vi "Setup Motors.vi"   [LabVIEW 2014]
uses:
  <vilib>/Rock Robotics/SystemInterfaces/DIO/FPGA_DIOPWMChannel.ctl
  <vilib>/Rock Robotics/SystemInterfaces/Typedef/FPGA_TypedefDigitalModule.ctl
  <vilib>/Rock Robotics/WPI/Joystick/WPI_JoystickDeviceEnum.ctl
  <vilib>/Rock Robotics/SystemInterfaces/Typedef/FPGA_TypedefAnalogModule.ctl
  <vilib>/Rock Robotics/SystemInterfaces/AI/FPGA_AIChannel.ctl
  <vilib>/Rock Robotics/WPI/Solenoid/WPI_SolenoidChannel.ctl
  <vilib>/Rock Robotics/SystemInterfaces/AI/FPGA_AIGyroChannel.ctl
  <vilib>/Rock Robotics/SystemInterfaces/Typedef/FPGA_TypedefAnalogModuleForGyro.ctl
  <vilib>/Rock Robotics/SystemInterfaces/DIO/FPGA_DIOChannel.ctl
  <vilib>/Rock Robotics/WPI/SafetyOutput/WPI_SafetyOutputConfigMenu.ctl
  <vilib>/Rock Robotics/WPI/MotorControl/WPI_MotorControlOpen Talon.vi
  <vilib>/Rock Robotics/WPI/Solenoid/WPI_SolenoidOpenSingle.vi
  <vilib>/Rock Robotics/WPI/Switch/WPI_SwitchOpenLimit.vi
  Global Variables.vi
types:
  T1 = typedef "WPI_SafetyOutputConfigMenu.ctl" = enum16{"Enable", "Disable"}
  T2 = typedef "FPGA_DIOChannel.ctl" = enum8{"DIO 0", "DIO 1", "DIO 2", "DIO 3", "DIO 4", "DIO 5", "DIO 6", "DIO 7", "DIO 8", "DIO 9", "DIO MXP 0", "DIO MXP 1", "DIO MXP 2", "DIO MXP 3", "DIO MXP 4", "DIO MXP 5", "DIO MXP 6", "DIO MXP 7", "DIO MXP 8", "DIO MXP 9", "DIO MXP 10", "DIO MXP 11", "DIO MXP 12", "DIO MXP 13", "DIO MXP 14", "DIO MXP 15", "Invalid"}
  T3 = typedef "FPGA_TypedefDigitalModule.ctl" = enum16{"Controller 1"}
  T4 = typedef "FPGA_TypedefAnalogModuleForGyro.ctl" = enum16{"Controller 1"}
  T5 = typedef "FPGA_AIGyroChannel.ctl" = enum8{"AI 0", "AI 1", "Invalid"}
  T6 = typedef "WPI_SolenoidChannel.ctl" = enum8{"Solenoid 0", "Solenoid 1", "Solenoid 2", "Solenoid 3", "Solenoid 4", "Solenoid 5", "Solenoid 6", "Solenoid 7", "Invalid"}
  T7 = typedef "FPGA_DIOPWMChannel.ctl" = enum8{"PWM 0", "PWM 1", "PWM 2", "PWM 3", "PWM 4", "PWM 5", "PWM 6", "PWM 7", "PWM 8", "PWM 9", "PWM MXP 0", "PWM MXP 1", "PWM MXP 2", "PWM MXP 3", "PWM MXP 4", "PWM MXP 5", "PWM MXP 6", "PWM MXP 7", "PWM MXP 8", "PWM MXP 9", "Invalid"}
  T8 = typedef "FPGA_AIChannel.ctl" = enum8{"AI 0", "AI 1", "AI 2", "AI 3", "AI MXP 0", "AI MXP 1", "AI MXP 2", "AI MXP 3", "Invalid"}
  T9 = typedef "FPGA_TypedefAnalogModule.ctl" = enum16{"Controller 1"}
  T10 = typedef "WPI_JoystickDeviceEnum.ctl" = enum16{"USB 0", "USB 1", "USB 2", "USB 3", "USB 4", "USB 5"}
  T11 = typedef "WPI_MotorControlDeviceRef.ctl" = cluster{"DeviceStatus":errorcluster, "Type":T12, "PWM":cluster{"Controller":T3, "PWM Channel":T7, "DeadBand":T13}, "CAN":cluster{"Device Number":u8, "Control Mode":T14, "Semaphore":T15, "Max Vout":dbl, "TalonSRX Control Mode":T16}, "Invert":bool, "TransformRef":T17, "InvTransformRef":T17}
  T12 = typedef "WPI_MotorControlType.ctl" = enum16{"PWM", "CAN", "CANTalonSRX"}
  T13 = typedef "WPI_PWMDeadband.ctl" = cluster{"Name":string, "maxPositivePwm":i32, "minPositivePwm":i32, "centerPwm":i32, "maxNegativePwm":i32, "minNegativePwm":i32, "angularRange":u16}
  T14 = typedef "WPI_CANJaguar_ControlMode.ctl" = enum8{"Percent VBus", "Current", "Speed", "Position", "Voltage"}
  T15 = typedef "Semaphore RefNum" = refnum<k1>
  T16 = typedef "WPI_CANTalonSRX_APIControlMode.ctl" = enum8{"Percent VBus", "Speed", "Position", "Slave", "Unchanged / Invalid"}
  T17 = typedef "WPI_PWMTransform_ConPane.ctl" = refnum<vi>
  T18 = typedef "WPI_GyroDevRef.ctl" = cluster{"DevStatus":errorcluster, "Analog Module":T9, "Analog Channel":T8, "Offset":dbl, "Gain (VoltsPerDegree/Second)":dbl}
  T19 = typedef "WPI_SolenoidDevRef.ctl" = cluster{"DevStatus":errorcluster, "Pneumatics Control Module":u8, "Forward Solenoid Channel":T6, "Reverse Solenoid Channel":T6}
  T20 = typedef "WPI_SwitchDevRef.ctl" = cluster{"DevStatus":errorcluster, "DIO Channel":T2, "Controller":T3, "CntIndex":T21, "Normally Closed":bool}
  T21 = typedef "FPGA_CounterCtrSystemIndex.ctl" = enum8{"Ctr 0", "Ctr 1", "Ctr 2", "Ctr 3", "Ctr 4", "Ctr 5", "Ctr 6", "Ctr 7", "Invalid"}
  T22 = typedef "WPI_AnalogChannelDevRef.ctl" = cluster{"DevStatus":errorcluster, "Controller":T9, "Analog Channel":T8}
  T23 = typedef "WPI_JoystickDevRef.ctl" = cluster{"Device":T10}
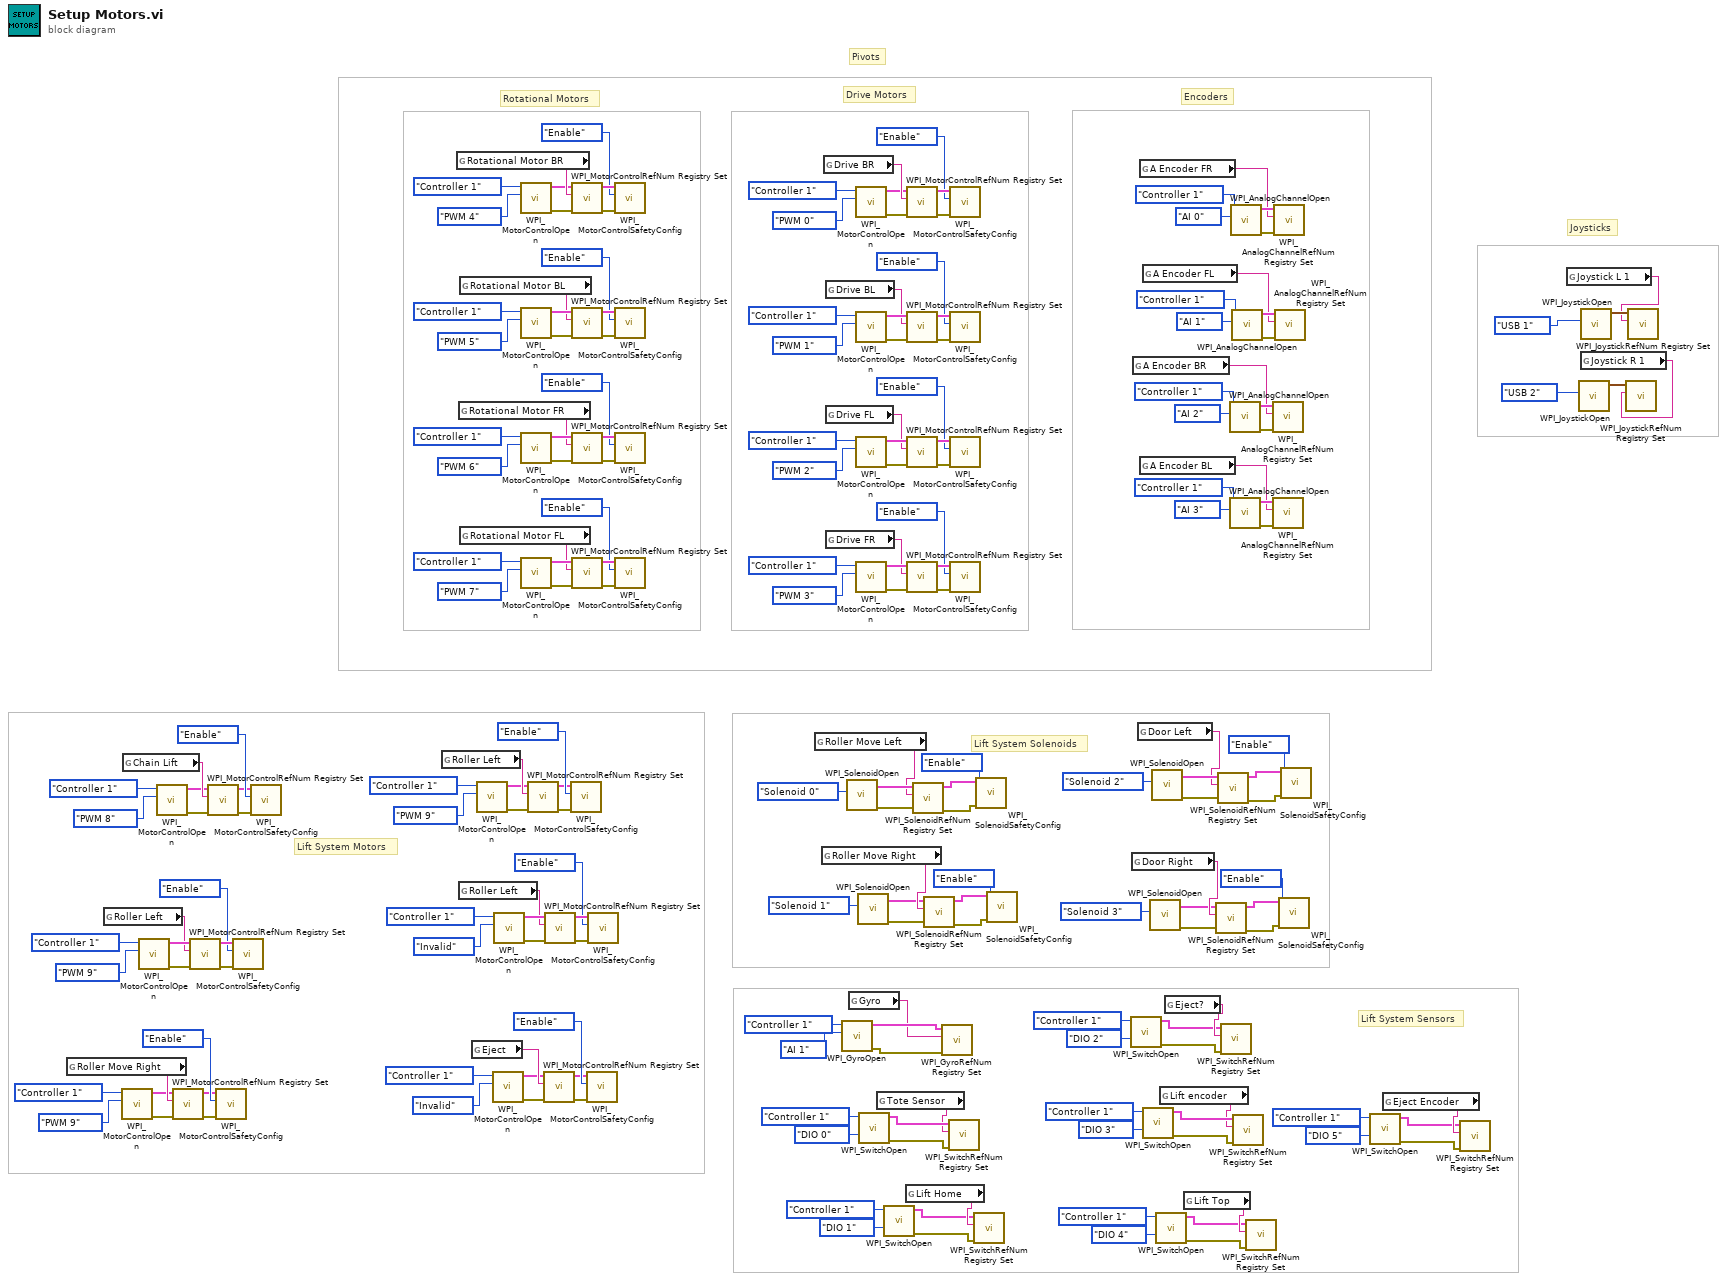
[diagram p0: block diagram]
diagram:
  # "Lift System Sensors"
  # "Lift System Solenoids"
  # "Lift System Motors"
  # "Encoders"
  # "Joysticks"
  # "Pivots"
  # "Rotational Motors"
  # "Drive Motors"
  n1 = global read "Global Variables.vi" "Roller Move Right"() -> (w94:string)
  n2 = global read "Global Variables.vi" "Roller Left"() -> (w97:string)
  n3 = call-poly <vilib>:"WPI_MotorControlOpen.vi"("PWM Channel"=FPGA_DIOPWMChannel."PWM 9", "Controller"=FPGA_TypedefDigitalModule."Controller 1") -> ("error out"=w89:errorcluster, "MotorControlDeviceRef"=w88:T11)  [unwired: 8 in]
  n4 = global read "Global Variables.vi" "Chain Lift"() -> (w110:string)
  n5 = call-poly <vilib>:"WPI_MotorControlOpen.vi"("PWM Channel"=FPGA_DIOPWMChannel."PWM 9", "Controller"=FPGA_TypedefDigitalModule."Controller 1") -> ("error out"=w102:errorcluster, "MotorControlDeviceRef"=w103:T11)  [unwired: 8 in]
  n6 = call-poly <vilib>:"WPI_MotorControlOpen.vi"("PWM Channel"=FPGA_DIOPWMChannel."PWM 8", "Controller"=FPGA_TypedefDigitalModule."Controller 1") -> ("error out"=w105:errorcluster, "MotorControlDeviceRef"=w104:T11)  [unwired: 8 in]
  n7 = call <vilib>:"WPI_MotorControlRefNum Registry Set.vi"("error in (no error)"=w89, "refnum name"=w94, "MotorControlDevRef"=w88) -> ("error out"=w91:errorcluster, "MotorControlDevRef"=w90:T11)  [unwired: 7 in]
  n8 = call <vilib>:"WPI_MotorControlRefNum Registry Set.vi"("error in (no error)"=w102, "refnum name"=w97, "MotorControlDevRef"=w103) -> ("error out"=w100:errorcluster, "MotorControlDevRef"=w101:T11)  [unwired: 7 in]
  n9 = call <vilib>:"WPI_MotorControlRefNum Registry Set.vi"("error in (no error)"=w105, "refnum name"=w110, "MotorControlDevRef"=w104) -> ("error out"=w107:errorcluster, "MotorControlDevRef"=w106:T11)  [unwired: 7 in]
  n10 = call <vilib>:"WPI_MotorControlSafetyConfig.vi"("error in (no error)"=w91, "mode"=WPI_SafetyOutputConfigMenu."Enable", "MotorControlDevRef"=w90) -> ()  [unwired: 7 in, 2 out]
  n11 = call <vilib>:"WPI_MotorControlSafetyConfig.vi"("error in (no error)"=w100, "mode"=WPI_SafetyOutputConfigMenu."Enable", "MotorControlDevRef"=w101) -> ()  [unwired: 7 in, 2 out]
  n12 = call <vilib>:"WPI_MotorControlSafetyConfig.vi"("error in (no error)"=w107, "mode"=WPI_SafetyOutputConfigMenu."Enable", "MotorControlDevRef"=w106) -> ()  [unwired: 7 in, 2 out]
  n13 = global read "Global Variables.vi" "Roller Left"() -> (w86:string)
  n14 = global read "Global Variables.vi" "Rotational Motor BR"() -> (w164:string)
  n15 = global read "Global Variables.vi" "Rotational Motor FR"() -> (w138:string)
  n16 = global read "Global Variables.vi" "Roller Left"() -> (w73:string)
  n17 = global read "Global Variables.vi" "Rotational Motor BL"() -> (w139:string)
  n18 = global read "Global Variables.vi" "Rotational Motor FL"() -> (w137:string)
  n19 = global read "Global Variables.vi" "Eject"() -> (w70:string)
  n20 = call-poly <vilib>:"WPI_MotorControlOpen.vi"("PWM Channel"=FPGA_DIOPWMChannel."PWM 9", "Controller"=FPGA_TypedefDigitalModule."Controller 1") -> ("error out"=w81:errorcluster, "MotorControlDeviceRef"=w80:T11)  [unwired: 8 in]
  n21 = call-poly <vilib>:"WPI_MotorControlOpen.vi"("PWM Channel"=FPGA_DIOPWMChannel."Invalid", "Controller"=FPGA_TypedefDigitalModule."Controller 1") -> ("error out"=w65:errorcluster, "MotorControlDeviceRef"=w64:T11)  [unwired: 8 in]
  n22 = call-poly <vilib>:"WPI_MotorControlOpen.vi"("PWM Channel"=FPGA_DIOPWMChannel."Invalid", "Controller"=FPGA_TypedefDigitalModule."Controller 1") -> ("error out"=w78:errorcluster, "MotorControlDeviceRef"=w79:T11)  [unwired: 8 in]
  n23 = call-poly <vilib>:"WPI_MotorControlOpen.vi"("PWM Channel"=FPGA_DIOPWMChannel."PWM 4", "Controller"=FPGA_TypedefDigitalModule."Controller 1") -> ("error out"=w162:errorcluster, "MotorControlDeviceRef"=w163:T11)  [unwired: 8 in]
  n24 = call-poly <vilib>:"WPI_MotorControlOpen.vi"("PWM Channel"=FPGA_DIOPWMChannel."PWM 5", "Controller"=FPGA_TypedefDigitalModule."Controller 1") -> ("error out"=w156:errorcluster, "MotorControlDeviceRef"=w157:T11)  [unwired: 8 in]
  n25 = call-poly <vilib>:"WPI_MotorControlOpen.vi"("PWM Channel"=FPGA_DIOPWMChannel."PWM 6", "Controller"=FPGA_TypedefDigitalModule."Controller 1") -> ("error out"=w150:errorcluster, "MotorControlDeviceRef"=w151:T11)  [unwired: 8 in]
  n26 = call-poly <vilib>:"WPI_MotorControlOpen.vi"("PWM Channel"=FPGA_DIOPWMChannel."PWM 7", "Controller"=FPGA_TypedefDigitalModule."Controller 1") -> ("error out"=w144:errorcluster, "MotorControlDeviceRef"=w145:T11)  [unwired: 8 in]
  n27 = call <vilib>:"WPI_MotorControlRefNum Registry Set.vi"("error in (no error)"=w81, "refnum name"=w86, "MotorControlDevRef"=w80) -> ("error out"=w83:errorcluster, "MotorControlDevRef"=w82:T11)  [unwired: 7 in]
  n28 = call <vilib>:"WPI_MotorControlRefNum Registry Set.vi"("error in (no error)"=w65, "refnum name"=w70, "MotorControlDevRef"=w64) -> ("error out"=w67:errorcluster, "MotorControlDevRef"=w66:T11)  [unwired: 7 in]
  n29 = call <vilib>:"WPI_MotorControlRefNum Registry Set.vi"("error in (no error)"=w78, "refnum name"=w73, "MotorControlDevRef"=w79) -> ("error out"=w76:errorcluster, "MotorControlDevRef"=w77:T11)  [unwired: 7 in]
  n30 = call <vilib>:"WPI_MotorControlSafetyConfig.vi"("error in (no error)"=w83, "mode"=WPI_SafetyOutputConfigMenu."Enable", "MotorControlDevRef"=w82) -> ()  [unwired: 7 in, 2 out]
  n31 = call <vilib>:"WPI_MotorControlRefNum Registry Set.vi"("error in (no error)"=w162, "refnum name"=w164, "MotorControlDevRef"=w163) -> ("error out"=w160:errorcluster, "MotorControlDevRef"=w161:T11)  [unwired: 7 in]
  n32 = call <vilib>:"WPI_MotorControlRefNum Registry Set.vi"("error in (no error)"=w156, "refnum name"=w139, "MotorControlDevRef"=w157) -> ("error out"=w154:errorcluster, "MotorControlDevRef"=w155:T11)  [unwired: 7 in]
  n33 = call <vilib>:"WPI_MotorControlRefNum Registry Set.vi"("error in (no error)"=w150, "refnum name"=w138, "MotorControlDevRef"=w151) -> ("error out"=w148:errorcluster, "MotorControlDevRef"=w149:T11)  [unwired: 7 in]
  n34 = call <vilib>:"WPI_MotorControlRefNum Registry Set.vi"("error in (no error)"=w144, "refnum name"=w137, "MotorControlDevRef"=w145) -> ("error out"=w142:errorcluster, "MotorControlDevRef"=w143:T11)  [unwired: 7 in]
  n35 = call <vilib>:"WPI_MotorControlSafetyConfig.vi"("error in (no error)"=w67, "mode"=WPI_SafetyOutputConfigMenu."Enable", "MotorControlDevRef"=w66) -> ()  [unwired: 7 in, 2 out]
  n36 = call <vilib>:"WPI_MotorControlSafetyConfig.vi"("error in (no error)"=w76, "mode"=WPI_SafetyOutputConfigMenu."Enable", "MotorControlDevRef"=w77) -> ()  [unwired: 7 in, 2 out]
  n37 = call <vilib>:"WPI_MotorControlSafetyConfig.vi"("error in (no error)"=w160, "mode"=WPI_SafetyOutputConfigMenu."Enable", "MotorControlDevRef"=w161) -> ()  [unwired: 7 in, 2 out]
  n38 = call <vilib>:"WPI_MotorControlSafetyConfig.vi"("error in (no error)"=w154, "mode"=WPI_SafetyOutputConfigMenu."Enable", "MotorControlDevRef"=w155) -> ()  [unwired: 7 in, 2 out]
  n39 = call <vilib>:"WPI_MotorControlSafetyConfig.vi"("error in (no error)"=w148, "mode"=WPI_SafetyOutputConfigMenu."Enable", "MotorControlDevRef"=w149) -> ()  [unwired: 7 in, 2 out]
  n40 = call <vilib>:"WPI_MotorControlSafetyConfig.vi"("error in (no error)"=w142, "mode"=WPI_SafetyOutputConfigMenu."Enable", "MotorControlDevRef"=w143) -> ()  [unwired: 7 in, 2 out]
  n41 = global read "Global Variables.vi" "Roller Move Left"() -> (w58:string)
  n42 = global read "Global Variables.vi" "Roller Move Right"() -> (w57:string)
  n43 = global read "Global Variables.vi" "Drive BR"() -> (w201:string)
  n44 = global read "Global Variables.vi" "Drive BL"() -> (w176:string)
  n45 = global read "Global Variables.vi" "Drive FL"() -> (w175:string)
  n46 = global read "Global Variables.vi" "Drive FR"() -> (w174:string)
  n47 = call <vilib>:"WPI_GyroOpen.vi"("Analog Channel"=FPGA_AIGyroChannel."AI 1", "Controller"=FPGA_TypedefAnalogModuleForGyro."Controller 1") -> ("error out"=w38:errorcluster, "GyroDevRef"=w39:T18)  [unwired: 7 in, 1 out]
  n48 = call-poly <vilib>:"WPI_SolenoidOpen.vi"("Solenoid Channel"=WPI_SolenoidChannel."Solenoid 0") -> ("error out"=w60:errorcluster, "SolenoidDevRef"=w61:T19)  [unwired: 9 in]
  n49 = global read "Global Variables.vi" "Gyro"() -> (w35:string)
  n50 = call-poly <vilib>:"WPI_MotorControlOpen.vi"("PWM Channel"=FPGA_DIOPWMChannel."PWM 0", "Controller"=FPGA_TypedefDigitalModule."Controller 1") -> ("error out"=w199:errorcluster, "MotorControlDeviceRef"=w200:T11)  [unwired: 8 in]
  n51 = call-poly <vilib>:"WPI_MotorControlOpen.vi"("PWM Channel"=FPGA_DIOPWMChannel."PWM 1", "Controller"=FPGA_TypedefDigitalModule."Controller 1") -> ("error out"=w193:errorcluster, "MotorControlDeviceRef"=w194:T11)  [unwired: 8 in]
  n52 = call-poly <vilib>:"WPI_MotorControlOpen.vi"("PWM Channel"=FPGA_DIOPWMChannel."PWM 2", "Controller"=FPGA_TypedefDigitalModule."Controller 1") -> ("error out"=w187:errorcluster, "MotorControlDeviceRef"=w188:T11)  [unwired: 8 in]
  n53 = call-poly <vilib>:"WPI_MotorControlOpen.vi"("PWM Channel"=FPGA_DIOPWMChannel."PWM 3", "Controller"=FPGA_TypedefDigitalModule."Controller 1") -> ("error out"=w181:errorcluster, "MotorControlDeviceRef"=w182:T11)  [unwired: 8 in]
  n54 = call-poly <vilib>:"WPI_SolenoidOpen.vi"("Solenoid Channel"=WPI_SolenoidChannel."Solenoid 1") -> ("error out"=w55:errorcluster, "SolenoidDevRef"=w54:T19)  [unwired: 9 in]
  n55 = call-poly <vilib>:"WPI_SwitchOpen.vi"("DIO Channel"=FPGA_DIOChannel."DIO 0", "Controller"=FPGA_TypedefDigitalModule."Controller 1") -> ("error out"=w33:errorcluster, "SwitchDevRef"=w34:T20)  [unwired: 8 in]
  n56 = global read "Global Variables.vi" "Tote Sensor"() -> (w30:string)
  n57 = call-poly <vilib>:"WPI_SwitchOpen.vi"("DIO Channel"=FPGA_DIOChannel."DIO 1", "Controller"=FPGA_TypedefDigitalModule."Controller 1") -> ("error out"=w26:errorcluster, "SwitchDevRef"=w25:T20)  [unwired: 8 in]
  n58 = global read "Global Variables.vi" "Lift Home"() -> (w29:string)
  n59 = call <vilib>:"WPI_MotorControlRefNum Registry Set.vi"("error in (no error)"=w199, "refnum name"=w201, "MotorControlDevRef"=w200) -> ("error out"=w197:errorcluster, "MotorControlDevRef"=w198:T11)  [unwired: 7 in]
  n60 = call <vilib>:"WPI_MotorControlRefNum Registry Set.vi"("error in (no error)"=w193, "refnum name"=w176, "MotorControlDevRef"=w194) -> ("error out"=w191:errorcluster, "MotorControlDevRef"=w192:T11)  [unwired: 7 in]
  n61 = call <vilib>:"WPI_MotorControlRefNum Registry Set.vi"("error in (no error)"=w187, "refnum name"=w175, "MotorControlDevRef"=w188) -> ("error out"=w185:errorcluster, "MotorControlDevRef"=w186:T11)  [unwired: 7 in]
  n62 = call <vilib>:"WPI_MotorControlRefNum Registry Set.vi"("error in (no error)"=w181, "refnum name"=w174, "MotorControlDevRef"=w182) -> ("error out"=w179:errorcluster, "MotorControlDevRef"=w180:T11)  [unwired: 7 in]
  n63 = call <vilib>:"WPI_SolenoidRefNum Registry Set.vi"("error in (no error)"=w60, "refnum name"=w58, "SolenoidDevRef"=w61) -> ("error out"=w62:errorcluster, "SolenoidDevRef"=w63:T19)  [unwired: 7 in]
  n64 = call <vilib>:"WPI_SolenoidRefNum Registry Set.vi"("error in (no error)"=w55, "refnum name"=w57, "SolenoidDevRef"=w54) -> ("error out"=w53:errorcluster, "SolenoidDevRef"=w52:T19)  [unwired: 7 in]
  n65 = call <vilib>:"WPI_GyroRefNum Registry Set.vi"("error in (no error)"=w38, "refnum name"=w35, "GyroDevRef"=w39) -> ()  [unwired: 7 in, 2 out]
  n66 = call <vilib>:"WPI_SwitchRefNum Registry Set.vi"("error in (no error)"=w33, "refnum name"=w30, "SwitchDevRef"=w34) -> ()  [unwired: 7 in, 2 out]
  n67 = call <vilib>:"WPI_MotorControlSafetyConfig.vi"("error in (no error)"=w197, "mode"=WPI_SafetyOutputConfigMenu."Enable", "MotorControlDevRef"=w198) -> ()  [unwired: 7 in, 2 out]
  n68 = call <vilib>:"WPI_MotorControlSafetyConfig.vi"("error in (no error)"=w191, "mode"=WPI_SafetyOutputConfigMenu."Enable", "MotorControlDevRef"=w192) -> ()  [unwired: 7 in, 2 out]
  n69 = call <vilib>:"WPI_MotorControlSafetyConfig.vi"("error in (no error)"=w185, "mode"=WPI_SafetyOutputConfigMenu."Enable", "MotorControlDevRef"=w186) -> ()  [unwired: 7 in, 2 out]
  n70 = call <vilib>:"WPI_MotorControlSafetyConfig.vi"("error in (no error)"=w179, "mode"=WPI_SafetyOutputConfigMenu."Enable", "MotorControlDevRef"=w180) -> ()  [unwired: 7 in, 2 out]
  n71 = call <vilib>:"WPI_SwitchRefNum Registry Set.vi"("error in (no error)"=w26, "refnum name"=w29, "SwitchDevRef"=w25) -> ()  [unwired: 7 in, 2 out]
  n72 = call <vilib>:"WPI_SolenoidSafetyConfig.vi"("error in (no error)"=w62, "mode"=WPI_SafetyOutputConfigMenu."Enable", "SolenoidDevRef"=w63) -> ()  [unwired: 7 in, 2 out]
  n73 = call <vilib>:"WPI_SolenoidSafetyConfig.vi"("error in (no error)"=w53, "mode"=WPI_SafetyOutputConfigMenu."Enable", "SolenoidDevRef"=w52) -> ()  [unwired: 7 in, 2 out]
  n74 = call-poly <vilib>:"WPI_SwitchOpen.vi"("DIO Channel"=FPGA_DIOChannel."DIO 2", "Controller"=FPGA_TypedefDigitalModule."Controller 1") -> ("error out"=w11:errorcluster, "SwitchDevRef"=w10:T20)  [unwired: 8 in]
  n75 = global read "Global Variables.vi" "Door Right"() -> (w45:string)
  n76 = global read "Global Variables.vi" "A Encoder BR"() -> (w113:string)
  n77 = global read "Global Variables.vi" "Door Left"() -> (w46:string)
  n78 = global read "Global Variables.vi" "A Encoder FR"() -> (w115:string)
  n79 = global read "Global Variables.vi" "A Encoder BL"() -> (w114:string)
  n80 = global read "Global Variables.vi" "A Encoder FL"() -> (w112:string)
  n81 = call-poly <vilib>:"WPI_SwitchOpen.vi"("DIO Channel"=FPGA_DIOChannel."DIO 3", "Controller"=FPGA_TypedefDigitalModule."Controller 1") -> ("error out"=w23:errorcluster, "SwitchDevRef"=w24:T20)  [unwired: 8 in]
  n82 = call-poly <vilib>:"WPI_SolenoidOpen.vi"("Solenoid Channel"=WPI_SolenoidChannel."Solenoid 3") -> ("error out"=w43:errorcluster, "SolenoidDevRef"=w42:T19)  [unwired: 9 in]
  n83 = call-poly <vilib>:"WPI_SolenoidOpen.vi"("Solenoid Channel"=WPI_SolenoidChannel."Solenoid 2") -> ("error out"=w48:errorcluster, "SolenoidDevRef"=w49:T19)  [unwired: 9 in]
  n84 = call-poly <vilib>:"WPI_SwitchOpen.vi"("DIO Channel"=FPGA_DIOChannel."DIO 4", "Controller"=FPGA_TypedefDigitalModule."Controller 1") -> ("error out"=w16:errorcluster, "SwitchDevRef"=w15:T20)  [unwired: 8 in]
  n85 = global read "Global Variables.vi" "Lift encoder"() -> (w20:string)
  n86 = global read "Global Variables.vi" "Eject?"() -> (w14:string)
  n87 = global read "Global Variables.vi" "Lift Top"() -> (w19:string)
  n88 = call <vilib>:"WPI_SolenoidRefNum Registry Set.vi"("error in (no error)"=w43, "refnum name"=w45, "SolenoidDevRef"=w42) -> ("error out"=w41:errorcluster, "SolenoidDevRef"=w40:T19)  [unwired: 7 in]
  n89 = call <vilib>:"WPI_SolenoidRefNum Registry Set.vi"("error in (no error)"=w48, "refnum name"=w46, "SolenoidDevRef"=w49) -> ("error out"=w50:errorcluster, "SolenoidDevRef"=w51:T19)  [unwired: 7 in]
  n90 = call <vilib>:"WPI_SwitchRefNum Registry Set.vi"("error in (no error)"=w11, "refnum name"=w14, "SwitchDevRef"=w10) -> ()  [unwired: 7 in, 2 out]
  n91 = call <vilib>:"WPI_AnalogChannelOpen.vi"("Analog Channel"=FPGA_AIChannel."AI 2", "Controller"=FPGA_TypedefAnalogModule."Controller 1") -> ("error out"=w122:errorcluster, "AIDeviceRef"=w123:T22)  [unwired: 8 in]
  n92 = call <vilib>:"WPI_AnalogChannelOpen.vi"("Analog Channel"=FPGA_AIChannel."AI 3", "Controller"=FPGA_TypedefAnalogModule."Controller 1") -> ("error out"=w118:errorcluster, "AIDeviceRef"=w119:T22)  [unwired: 8 in]
  n93 = call <vilib>:"WPI_AnalogChannelOpen.vi"("Analog Channel"=FPGA_AIChannel."AI 0", "Controller"=FPGA_TypedefAnalogModule."Controller 1") -> ("error out"=w130:errorcluster, "AIDeviceRef"=w131:T22)  [unwired: 8 in]
  n94 = call <vilib>:"WPI_AnalogChannelOpen.vi"("Analog Channel"=FPGA_AIChannel."AI 1", "Controller"=FPGA_TypedefAnalogModule."Controller 1") -> ("error out"=w126:errorcluster, "AIDeviceRef"=w127:T22)  [unwired: 8 in]
  n95 = call <vilib>:"WPI_SwitchRefNum Registry Set.vi"("error in (no error)"=w23, "refnum name"=w20, "SwitchDevRef"=w24) -> ()  [unwired: 7 in, 2 out]
  n96 = call <vilib>:"WPI_SwitchRefNum Registry Set.vi"("error in (no error)"=w16, "refnum name"=w19, "SwitchDevRef"=w15) -> ()  [unwired: 7 in, 2 out]
  n97 = call <vilib>:"WPI_AnalogChannelRefNum Registry Set.vi"("error in (no error)"=w122, "refnum name"=w113, "AIDeviceRef"=w123) -> ()  [unwired: 7 in, 2 out]
  n98 = call <vilib>:"WPI_AnalogChannelRefNum Registry Set.vi"("error in (no error)"=w118, "refnum name"=w114, "AIDeviceRef"=w119) -> ()  [unwired: 7 in, 2 out]
  n99 = call <vilib>:"WPI_AnalogChannelRefNum Registry Set.vi"("error in (no error)"=w130, "refnum name"=w115, "AIDeviceRef"=w131) -> ()  [unwired: 7 in, 2 out]
  n100 = call <vilib>:"WPI_AnalogChannelRefNum Registry Set.vi"("error in (no error)"=w126, "refnum name"=w112, "AIDeviceRef"=w127) -> ()  [unwired: 7 in, 2 out]
  n101 = call <vilib>:"WPI_SolenoidSafetyConfig.vi"("error in (no error)"=w41, "mode"=WPI_SafetyOutputConfigMenu."Enable", "SolenoidDevRef"=w40) -> ()  [unwired: 7 in, 2 out]
  n102 = call <vilib>:"WPI_SolenoidSafetyConfig.vi"("error in (no error)"=w50, "mode"=WPI_SafetyOutputConfigMenu."Enable", "SolenoidDevRef"=w51) -> ()  [unwired: 7 in, 2 out]
  n103 = call-poly <vilib>:"WPI_SwitchOpen.vi"("DIO Channel"=FPGA_DIOChannel."DIO 5", "Controller"=FPGA_TypedefDigitalModule."Controller 1") -> ("error out"=w6:errorcluster, "SwitchDevRef"=w5:T20)  [unwired: 8 in]
  n104 = global read "Global Variables.vi" "Eject Encoder"() -> (w9:string)
  n105 = call <vilib>:"WPI_SwitchRefNum Registry Set.vi"("error in (no error)"=w6, "refnum name"=w9, "SwitchDevRef"=w5) -> ()  [unwired: 7 in, 2 out]
  n106 = global read "Global Variables.vi" "Joystick L 1"() -> (w168:string)
  n107 = call <vilib>:"WPI_JoystickOpen.vi"("JoystickDevice"=WPI_JoystickDeviceEnum."USB 2") -> ("JoystickDevRef"=w166:T23)  [unwired: 10 in]
  n108 = call <vilib>:"WPI_JoystickOpen.vi"("JoystickDevice"=WPI_JoystickDeviceEnum."USB 1") -> ("JoystickDevRef"=w169:T23)  [unwired: 10 in]
  n109 = global read "Global Variables.vi" "Joystick R 1"() -> (w165:string)
  n110 = call <vilib>:"WPI_JoystickRefNum Registry Set.vi"("refnum name"=w165, "JoystickDevRef"=w166) -> ()  [unwired: 8 in, 2 out]
  n111 = call <vilib>:"WPI_JoystickRefNum Registry Set.vi"("refnum name"=w168, "JoystickDevRef"=w169) -> ()  [unwired: 8 in, 2 out]
